vi "generate default line.vi"(8 "error in":errorcluster, 11 "objects in":T1) -> (0 "error out":errorcluster, 2 "Line":T2, 3 "objects out":T1)   [LabVIEW 2020, in "DDS editor node.lvclass"]
uses:
  dds editor node.lvclass
  module/configuration/Line.ctl
  <vilib>/NI/Tag Bus Module Framework/channel/TBM channel.lvclass
  C:/Program Files (x86)/National Instruments/LabVIEW 2020/vi.lib/NI/Tag Bus/tag/tag descriptor.lvclass
  <vilib>/RTI DDS Toolkit/Types/RTI DDS Advanced Reader Configuration.ctl
  <vilib>/NI/DCAF/Tag Editor Core/Table API/Table Manager/object ref.ctl
  <vilib>/NI/DCAF/Tag Editor Core/Configuration Editor/Classes/Engine Parent/Engine Parent Editor Node.lvclass
  <vilib>/NI/DCAF/Tag Editor Core/Configuration Editor/Classes/Module editor node/module editor node.lvclass
  C:/Program Files (x86)/National Instruments/LabVIEW 2020/vi.lib/NI/Configuration Framework/serializable node/NISE_CEF_serializable node.lvclass
  <vilib>/NI/Tag Bus/tag/Data Type.ctl
  permissions.ctl
  module/configuration/dds configuration.lvclass
  <vilib>/NI/Tag Bus/tag/tag descriptor.lvclass/tag descriptor.ctl
  <vilib>/NI/Tag Bus/tag/read tag name.vi
  <vilib>/NI/Configuration Framework/serializable configuration/NISE_CEF_serializable configuration.lvclass
  <vilib>/NI/Tag Bus/tag/tag descriptor.lvclass
  <vilib>/RTI DDS Toolkit/Library/LVDDS_library.lvlib
  <vilib>/NI/DCAF/Tag Editor Core/Table API/Table Manager/Table Manager.lvclass
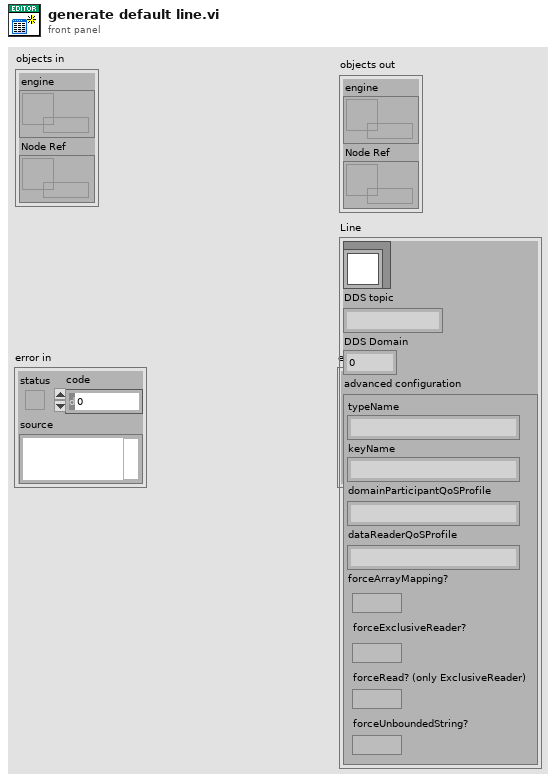
[diagram p1: front panel]
types:
  T1 = typedef "Table Manager.lvlib/Table Manager.lvclass/object ref.ctl" = cluster{"engine":refnum<data-value>, "Node Ref":refnum<data-value>}
  T2 = typedef "DDS configuration.lvclass/Line.ctl" = cluster{"channel":refnum<class "TBM channel.lvclass">, "DDS topic":string, "DDS Domain":u32, "advanced configuration":T3}
  T3 = typedef "LVDDS_library.lvlib/RTI DDS Advanced Reader Configuration.ctl" = cluster{"typeName":string, "keyName":string, "domainParticipantQoSProfile":string, "dataReaderQoSProfile":string, "forceArrayMapping?":bool, "forceExclusiveReader?":bool, "forceRead? (only ExclusiveReader)":bool, "forceUnboundedString?":bool}
  T4 = typedef "DDS editor node.lvclass/permissions.ctl" = enum32{"Read from DDS", "Write to DDS"}
  T5 = typedef "tag bus.lvlib/tag descriptor.lvclass/Data Type.ctl" = enum16{"Double", "Single", "I64", "I32", "I16", "I8", "U64", "U32", "U16", "U8", "Boolean", "String", "Array of Double", "Array of Single", "Array of I64", "Array of I32", "Array of I16", "Array of I8", "Array of U64", "Array of U32", "Array of U16", "Array of U8", "Array of Boolean", "Array of String"}
  T6 = typedef "TBM channel.lvclass/channel classification.ctl" = enum16{"input data", "output data", "processing parameter", "processing result"}
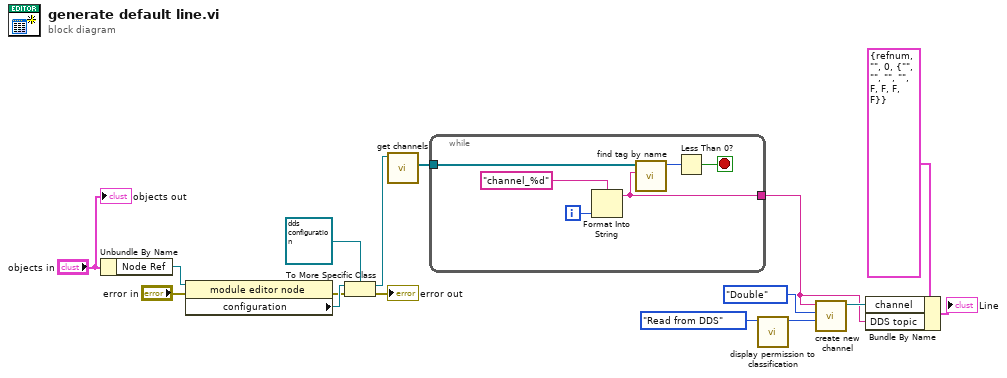
[diagram p0: block diagram]
diagram:
  n1 = Unbundle By Name("objects in") -> ("Node Ref"=w11:refnum<data-value>)
  n2 = property class="module editor node"(reference=w11, error in="error in") -> (error out=w5:errorcluster, "configuration"=w10:refnum<class "NISE_CEF_serializable configuration.lvclass">)  [unwired: 1 out]
  n3 = To More Specific Class(target class=refnum<class "dds configuration.lvclass"> refnum ("module configuration in"), reference=w10, error in=w5) -> (specific class reference=w9:refnum<class "dds configuration.lvclass">, error out=→"error out":errorcluster)
  n4 = call-dynamic "get channels.vi"("dds configuration in"=w9) -> ("channels"=w7:refnum<class "TBM channel.lvclass">[])  [unwired: 9 in, 1 out]
  n5 = while {
    tunnel: [w19] -> w1
    tunnel: w7 -> [w20]
    i -> [w22]
    stop <- w17 stop-if-true
    n6 = Format Into String(format string="channel_%d", w22) -> (resulting string=w19:string)  [unwired: 2 in, 1 out]
    n7 = call <vilib>:"find tag by name.vi"("name"=w19, "tags in"=w20) -> ("index"=w18:i32)  [unwired: 9 in]
    n8 = Less Than 0?(x=w18) -> (x < 0?=w17:bool)
  }
  n9 = call "display permission to classification.vi"("display permissions"=permissions."Read from DDS") -> ("channel classification"=w12:T6)  [unwired: 10 in]
  n10 = call <vilib>:"create new channel.vi"("channel classification"=w12, "data type"=Data_Type."Double", "channel name"=w1) -> ("channel"=w15:refnum<class "TBM channel.lvclass">)  [unwired: 8 in]
  n11 = Bundle By Name(cluster=T2 {"channel"=refnum, "DDS topic"="", "DDS Domain"=0, "advanced configuration"={"typeName"="", "keyName"="", "domainParticipantQoSProfile"="", "dataReaderQoSProfile"="", "forceArrayMapping?"=FALSE, "forceExclusiveReader?"=FALSE, "forceRead? (only ExclusiveReader)"=FALSE, "forceUnboundedString?"=FALSE}} ("Line"), "channel"=w15, "DDS topic"=w1) -> (→"Line":T2)
  "objects out" <- "objects in"
